vi "XY Graph Interpolate Plot Event.vi"(8 "Error In":errorcluster, 11 "Mouse Click Event Data":T1) -> (0 "Error Out":errorcluster, 1 "Message":string, 3 "Plot Name":string, 5 "Graph Name":string)   [LabVIEW 2019, in "XY Graph Add-Ons.lvlib"]
uses:
  XY Graph Add-Ons.lvlib
  XY Graph Mouse Click Event Data.ctl
  XY Graph Refnum.ctl
  <vilib>/Utility/miscctls.llb/LVPoint32TypeDef.ctl
  <vilib>/addons/_Advanced Signal Processing/NI_AdvSigProcTSA.lvlib
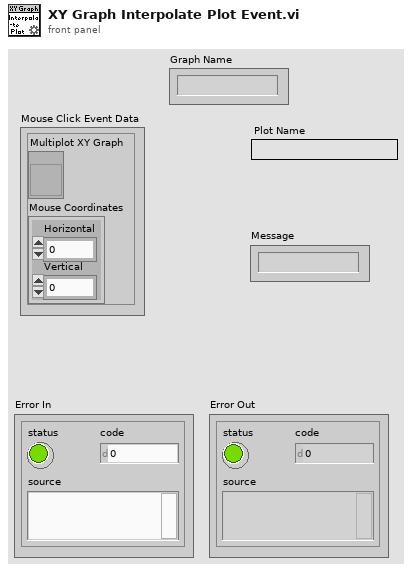
[diagram p1: front panel]
types:
  T1 = typedef "XY Graph Add-Ons.lvlib/XY Graph Mouse Click Event Data.ctl" = cluster{"Multiplot XY Graph":T2, "Mouse Coordinates":T3}
  T2 = typedef "XY Graph Add-Ons.lvlib/XY Graph Refnum.ctl" = refnum<vi>
  T3 = typedef "LVPoint32TypeDef.ctl" = cluster{"Horizontal":i32, "Vertical":i32}
  T4 = cluster{"Xt resampled":dbl[], "Xt resampled":dbl[]}
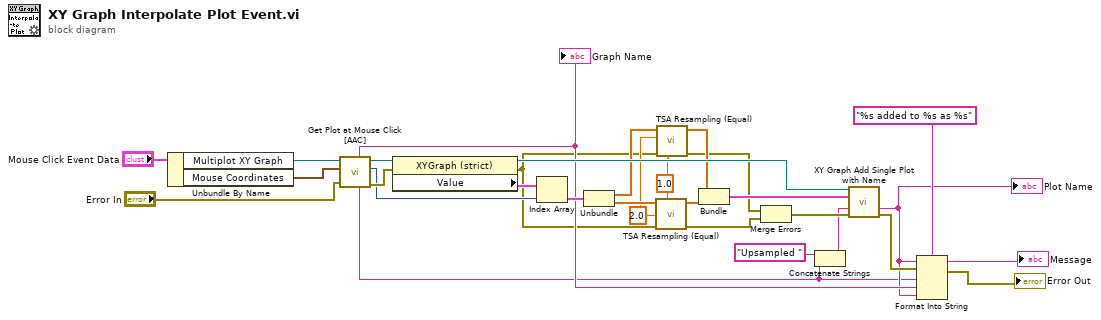
[diagram p0: block diagram]
diagram:
  w9 = 2.0 ("new sampling rate")
  w8 = 1.0 ("original sampling rate")
  n1 = Unbundle By Name("Mouse Click Event Data") -> ("Multiplot XY Graph"=w29:T2, "Mouse Coordinates"=w28:T3)
  n2 = call "Get Plot at Mouse Click [AAC].vi"("error in (no error)"="Error In", "Mouse Click Coordinates"=w28, "XYGraph Ref"=w29) -> ("error out"=w25:errorcluster, "Plot at Coordinates"=w23:i32, "XYGraph Ref"=w26:T2, "Plot Name"=w2:string, "Graph Name"=w12:string)  [unwired: 2 in, 2 out]
  "Graph Name" <- w12
  n3 = property class="XYGraph (strict)"(reference=w26, error in=w25) -> (reference out=w21:T2, error out=w7:errorcluster, "Value"=w24:cluster{"X Array":dbl[], "Y Array":dbl[]}[])
  n4 = Index Array(array=w24, index=w23) -> (element=w22:cluster{"X Array":dbl[], "Y Array":dbl[]})
  n5 = Unbundle(w22) -> ("X Array"=w10:dbl[], "Y Array"=w16:dbl[])
  n6 = call <vilib>:"TSA Resampling (Equal).vi"("original sampling rate"=w8, "error in (no error)"=w7, "new sampling rate"=w9, "Xt"=w16) -> ("error out"=w14:errorcluster, "Xt resampled"=w15:dbl[])  [unwired: 6 in]
  n7 = call <vilib>:"TSA Resampling (Equal).vi"("original sampling rate"=w8, "error in (no error)"=w7, "new sampling rate"=w9, "Xt"=w10) -> ("error out"=w4:errorcluster, "Xt resampled"=w6:dbl[])  [unwired: 6 in]
  n8 = Bundle("Xt resampled"=w6, "Xt resampled"=w15) -> (w13:T4)  [unwired: 1 in]
  n9 = Merge Errors(w4, w14) -> (w5:errorcluster)
  n10 = Concatenate Strings("Upsampled " ("format string"), w2) -> (w1:string)
  n11 = call "XY Graph Add Single Plot with Name.vi"("XYGraph Ref in"=w21, "Plot"=w13, "Plot Name (\"Plot\")"=w1, "error in (no error)"=w5) -> ("Plot Name"=w11:string, "error out"=w17:errorcluster)  [unwired: 8 in, 2 out]
  "Plot Name" <- w11
  n12 = Format Into String(format string="%s added to %s as %s", initial string=w11, error in=w17, w2, w12, w11) -> (resulting string=→"Message":string, error out=→"Error Out":errorcluster)
